vi "MSScript_Transform_Extended.vi"(5 "upper limit (Inf)":ext=inf format="%#_13g", 7 "lower limit (-Inf)":ext=-inf, 11 "Check_Str":string) -> (1 "Is a variable ?":bool, 2 "Value Error?":bool, 3 "Value Output":ext)   [LabVIEW 2018, in "MSScript.lvclass"]
uses:
  MSScript.lvclass
  <vilib>/regexp/Match Regular Expression.xnode
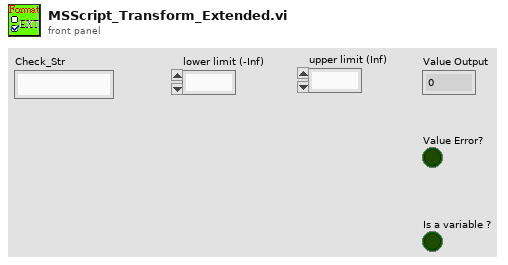
[diagram p1: front panel]
types:
  T1 = enum16{"Scalar", "ScalarArray", "Var", "VarArray", "Error"}
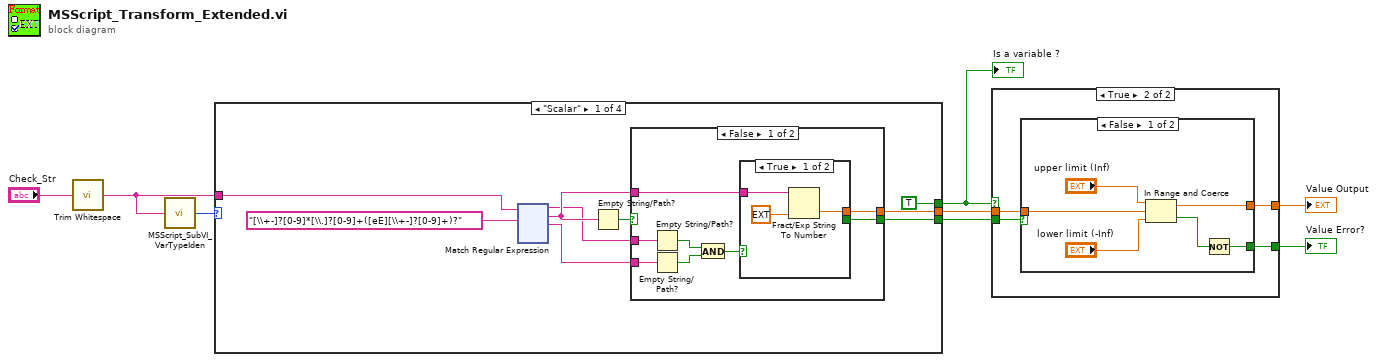
[diagram p0: block diagram]
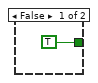
[diagram p2: hidden frame]
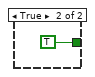
[diagram p3: hidden frame]
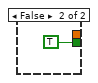
[diagram p4: hidden frame]
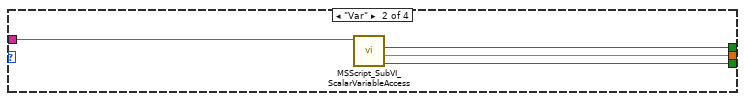
[diagram p6: hidden frame]
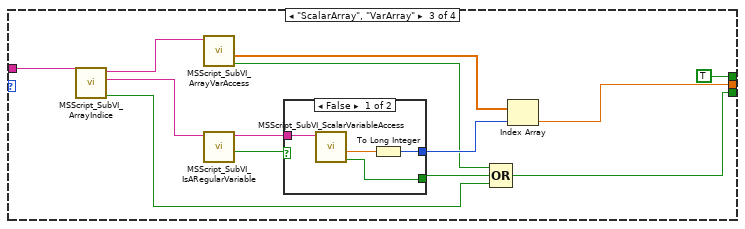
[diagram p7: hidden frame]
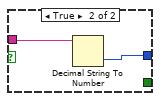
[diagram p8: hidden frame]
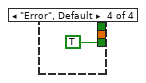
[diagram p9: hidden frame]
diagram:
  n1 = call <vilib>:"Trim Whitespace.vi"("string"="Check_Str") -> ("trimmed string"=w2:string)  [unwired: 1 in]
  n2 = call "MSScript_SubVI_VarTypeIden.vi"("Var in"=w2) -> ("Type"=w1:T1)
  n3 = case shown="\"Scalar\"" w1 {
    tunnel: [w16 w145 w150 TRUE ("Error?")] -> w6
    tunnel: [w15 w147 w154 _] -> w5
    tunnel: w2 -> [w10 w148 w161 _]
    tunnel: [TRUE ("Is a variable ?") w146 TRUE ("Is a variable ?") _] -> w7
    frame "Scalar" {
      n4 = xnode "Match Regular Expression"("input string"=w10, "regular expression"="[\\+-]?[0-9]*[\\.]?[0-9]+([eE][\\+-]?[0-9]+)?") -> ("before match"=w11:string, "whole match"=w12:string, "after match"=w13:string)  [unwired: 4 in, 2 out]
      n5 = Empty String/Path?(string/path=w12) -> (empty?=w17:bool)
      n6 = case shown="False" w17 {
        selector: w17 -> [_ w144]
        tunnel: [w134 w144] -> w16
        tunnel: w11 -> [w136 _]
        tunnel: w13 -> [w137 _]
        tunnel: w12 -> [w133 _]
        tunnel: [w132 _] -> w15
        frame False {
          n7 = Empty String/Path?(string/path=w136) -> (empty?=w138:bool)
          n8 = Empty String/Path?(string/path=w137) -> (empty?=w139:bool)
          n9 = And(x=w138, y=w139) -> (x .and. y?=w135:bool)
          n10 = case shown="True" w135 {
            tunnel: [_ TRUE] -> w134
            tunnel: w133 -> [w142 _]
            tunnel: [w140 _] -> w132
            frame True {
              n11 = Fract/Exp String To Number(string=w142, default (0 dbl)=ext 0.0) -> (number=w140:ext)  [unwired: 2 in, 1 out]
            }
            frame False {
            }
          }
        }
        frame True {
        }
      }
    }
    frame "Var" {
      n12 = call "MSScript_SubVI_ScalarVariableAccess.vi"("VarName"=w148) -> ("Value Error?"=w145:bool, "OutputValue"=w147:ext, "Is a variable ?"=w146:bool)  [unwired: 6 in]
    }
    frame "ScalarArray", "VarArray" {
      n13 = call "MSScript_SubVI_ArrayIndice.vi"("@name[x:y|z]"=w161) -> ("Index no found"=w149:bool, "Indice string"=w159:string, "@name"=w160:string)  [unwired: 6 in]
      n14 = call "MSScript_SubVI_ArrayVarAccess.vi"("VarName"=w160) -> ("Value Error?"=w151:bool, "ArrayVariable out"=w156:ext[])  [unwired: 6 in, 1 out]
      n15 = call "MSScript_SubVI_IsARegularVariable.vi"("VarString in"=w159) -> ("Variable simbol no found"=w158:bool, "VarString out"=w157:string)  [unwired: 6 in, 1 out]
      n16 = case shown="False" w158 {
        tunnel: w157 -> [w165 w167]
        tunnel: [w163 w166] -> w155
        tunnel: [w162 _] -> w152
        frame False {
          n17 = call "MSScript_SubVI_ScalarVariableAccess.vi"("VarName"=w165) -> ("Value Error?"=w162:bool, "OutputValue"=w164:ext)  [unwired: 6 in, 1 out]
          n18 = To Long Integer(number=w164) -> (32bit integer=w163:i32)
        }
        frame True {
          n19 = Decimal String To Number(string=w167) -> (number=w166:i32)  [unwired: 2 in, 1 out]
        }
      }
      n20 = Compound Arithmetic op=OR(w151, w152, w149) -> (w150:bool)
      n21 = Index Array(array=w156, index=w155) -> (element=w154:ext)
    }
    frame "Error", Default {
    }
  }
  "Is a variable ?" <- w7
  n22 = case shown="True" w7 {
    tunnel: w6 -> [_ w173]
    tunnel: w5 -> [_ w171]
    tunnel: [TRUE w172] -> w4
    tunnel: [_ w170] -> w3
    frame False {
    }
    frame True {
      n23 = case shown="False" w173 {
        tunnel: [w174 TRUE] -> w172
        tunnel: w171 -> [w177 _]
        tunnel: [w176 _] -> w170
        frame False {
          n24 = In Range and Coerce(upper limit="upper limit (Inf)", x=w177, lower limit="lower limit (-Inf)") -> (coerced(x)=w176:ext, In Range?=w175:bool)
          n25 = Not(x=w175) -> (.not. x?=w174:bool)
        }
        frame True {
        }
      }
    }
  }
  "Value Error?" <- w4
  "Value Output" <- w3
